vi "Clear Steps.vi"(8 "error in (no error)":errorcluster, 11 "Actor in":refnum<class "Actor.lvclass">) -> (0 "error out":errorcluster, 3 "Actor out":refnum<class "Actor.lvclass">)   [LabVIEW 2015, in "Actor.lvclass"]
uses:
  Actor.lvclass
  Actor.lvclass/Actor.ctl
  Sequencer/Sequencer.lvclass
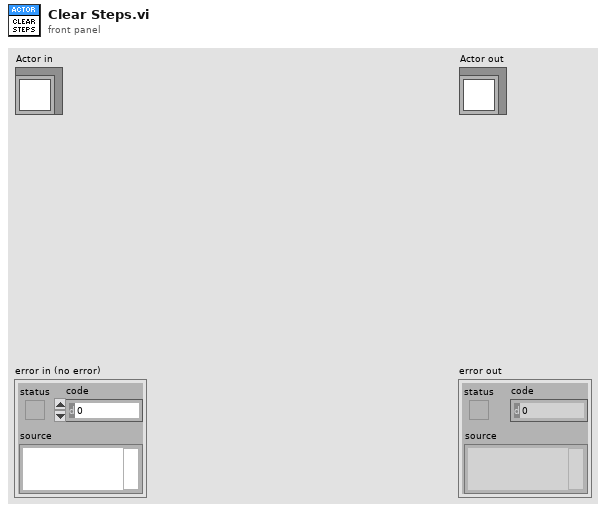
[diagram p1: front panel]
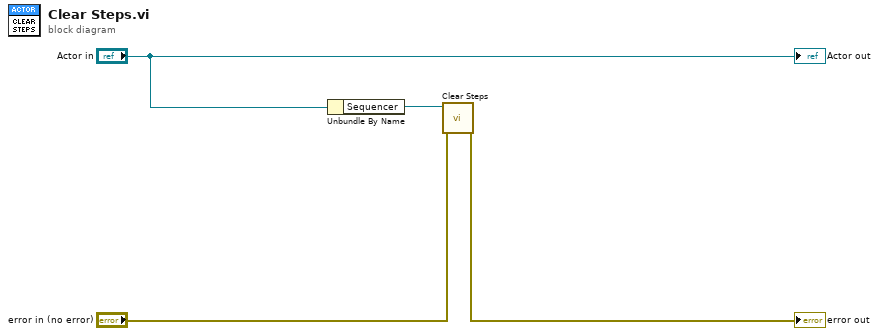
[diagram p0: block diagram]
diagram:
  n1 = Unbundle By Name("Actor in") -> ("Sequencer"=w1:refnum<class "Sequencer.lvclass">)
  n2 = call "Clear Steps.vi"("error in (no error)"="error in (no error)", "Sequencer in"=w1) -> ("error out"=→"error out":errorcluster)  [unwired: 9 in]
  "Actor out" <- "Actor in"
